vi "getLineImage.vi"(10 "Image In":T1, 11 "IMAQ Session In":refnum<k11>) -> (0 "IMAQ Session Out":refnum<k11>, 3 "Image Out":T1)   [LabVIEW 2011]
uses:
  <vilib>/vision/Image Controls.llb/IMAQ Image.ctl
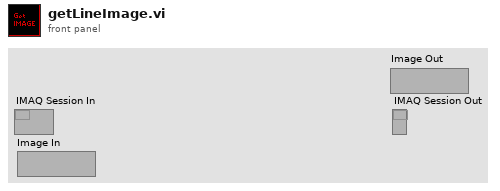
[diagram p1: front panel]
types:
  T1 = typedef "IMAQ Image.ctl" = refnum<image>
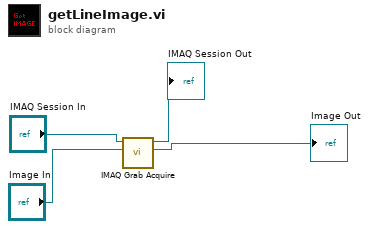
[diagram p0: block diagram]
diagram:
  n1 = call <vilib>:"IMAQ Grab Acquire.vi"("Image In"="Image In", "IMAQ Session In"="IMAQ Session In") -> ("Image Out"=→"Image Out":T1, "IMAQ Session Out"=→"IMAQ Session Out":refnum<k11>)  [unwired: 6 in, 2 out]
